vi "SRS PTC10 Read.vi"(2 "Point #":i32, 3 "Parameters":dbl[](array[numeric]) format="%.3e", 4 "Instrument Address":refnum<visa-resource-name>) -> (0 "Stop":bool, 1 "Measurement":dbl[](array[numeric]) format="%.6e")   [LabVIEW 2019]
doc: "This VI reads a single reading from a LakeShore 340 Temperature Controller. The stop boolean is always false. If no reading is obtained a single zero is returned.\nParameter 0 - 0=Resistance, 1=Temperature, 2=Heater Power\nParameter 1 - Channel to read, channel 0 is channel A, etc.\nScott Hannahs, <sth@magnet.fsu.edu> NHMFL-FSU, May 2003"
panel:
  # "The first parameter tells it\nCard Slot (1,2 or 5)\nThe second is channel #\n(1=A, 2=B...)"
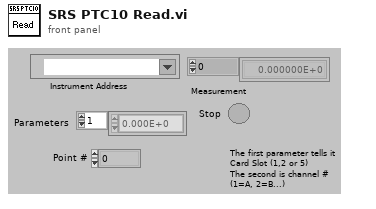
[diagram p1: front panel]
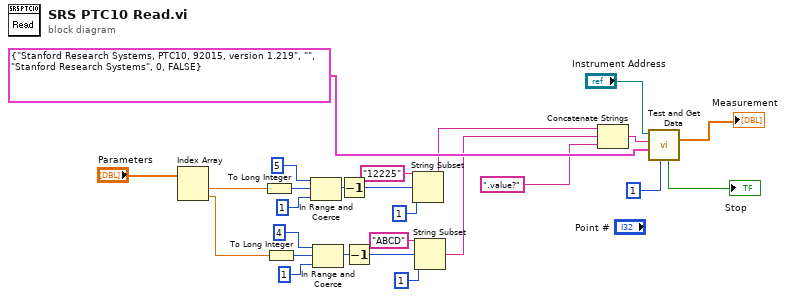
[diagram p0: block diagram]
diagram:
  n1 = Index Array(array="Parameters") -> (element #1=w14:dbl, element #2=w7:dbl)  [unwired: 2 in]
  n2 = To Long Integer(number=w14) -> (32bit integer=w19:i32)
  n3 = To Long Integer(number=w7) -> (32bit integer=w11:i32)
  n4 = In Range and Coerce(upper limit=5, x=w19, lower limit=1) -> (coerced(x)=w16:i32)  [unwired: 1 out]
  n5 = In Range and Coerce(upper limit=4, x=w11, lower limit=1) -> (coerced(x)=w8:i32)  [unwired: 1 out]
  n6 = Decrement(x=w16) -> (x-1=w5:i32)
  n7 = Decrement(x=w8) -> (x-1=w6:i32)
  n8 = String Subset(string="12225", offset (0)=w5, length (rest)=1 ("length (rest)")) -> (substring=w4:string)
  n9 = String Subset(string="ABCD", offset (0)=w6, length (rest)=1 ("length (rest)")) -> (substring=w3:string)
  n10 = Concatenate Strings(w4, w3, ".value?" ("string")) -> (w22:string)
  n11 = call "Test and Get Data.vi"("Point #"=1, "Instrument Info"=cluster{string, string, string, u32, bool} {"Stanford Research Systems, PTC10, 92015, version 1.219", "", "Stanford Research Systems", 0, FALSE}, "Command String"=w22, "VISA Sesson"="Instrument Address") -> ("Measurement"=→"Measurement":dbl[], "Stop"=→"Stop":bool)  [unwired: 2 in, 3 out]
